vi "SetFPGActrlParams_v2.vi"(4 "Twist Lead":T3={"Twist Lead Num (a0,a1)"=[60.0, 120.0, 120.0], "Twist Lead Den (b0,b1)"=[60.0, 120.0, 120.0]} {"Twist Lead Den (b0,b1)" format="%#_5e"; "Twist Lead Num (a0,a1)" format="%#_5e"}, 5 "Notch":T2={"Bend"={"Notch Num (a0,a1,a2)"=[60.0, 120.0, 120.0], "Notch Den (b0,b1)"=[60.0, 120.0, 120.0]}, "Twist"={"Notch Num (a0,a1,a2)"=[60.0, 120.0, 120.0], "Notch Den (b0,b1)"=[60.0, 120.0, 120.0]}} {"Twist"."Notch Den (b0,b1)" format="%#_5e"; "Twist"."Notch Num (a0,a1,a2)" format="%#_5e"; "Bend"."Notch Den (b0,b1)" format="%#_5e"; "Bend"."Notch Num (a0,a1,a2)" format="%#_5e"}, 6 "Bend Lead":T4={"Bend Lead Num (a1,a2)"=[60.0, 120.0, 120.0], "Bend Lead Den (b0,b1)"=[60.0, 120.0, 120.0]} {"Bend Lead Den (b0,b1)" format="%#_5e"; "Bend Lead Num (a1,a2)" format="%#_5e"}, 7 "Run Controller?":bool, 8 "error in (no error)":errorcluster, 9 "Ki*Ts":T1=[120.0, 60.0, 60.0], 10 "Kp":T5=[10000.0, 10000000.0, 10000000.0] format="%#_5g", 11 "FPGA VI Reference In":T6) -> (0 "error out":errorcluster, 3 "FPGA VI Reference Out":T6)   [LabVIEW 2017]
doc: "Pass parameters to FPGA:\n- Run controller?\n- Kp\n- Ki\n- tau, w0 (lead)\n- LPF_omega"
uses:
  <vilib>/rvi/interface/nirviReadWriteControl/nirviReadWriteControl.xnode
  TypeDefs/FPGA VI Reference.ctl
  FPGA Bitfiles/flexlab_FPGATarget_Tbeam256MAMainVI_XFHOL9u-69o.lvbitx
  NiFpgaLv.dll
  <vilib>/Utility/error.llb/Error Cluster From Error Code.vi
  <vilib>/rvi/errors/niLvFpgaAdjustHostInterfaceError.vi
  TypeDefs/Kp.ctl
  TypeDefs/Ki.ctl
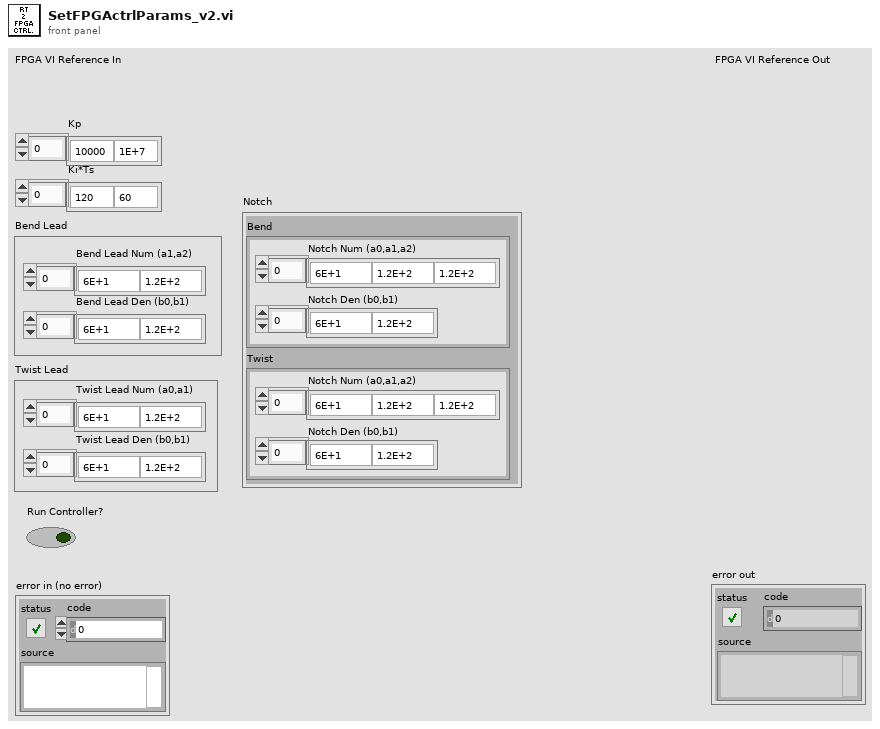
[diagram p1: front panel]
types:
  T1 = typedef "Ki.ctl" = dbl[]
  T2 = cluster{"Bend":cluster{"Notch Num (a0,a1,a2)":T1, "Notch Den (b0,b1)":T1}, "Twist":cluster{"Notch Num (a0,a1,a2)":T1, "Notch Den (b0,b1)":T1}}
  T3 = cluster{"Twist Lead Num (a0,a1)":T1, "Twist Lead Den (b0,b1)":T1}
  T4 = cluster{"Bend Lead Num (a1,a2)":T1, "Bend Lead Den (b0,b1)":T1}
  T5 = typedef "Kp.ctl" = dbl[]
  T6 = typedef "FPGA VI Reference.ctl" = refnum<k20>
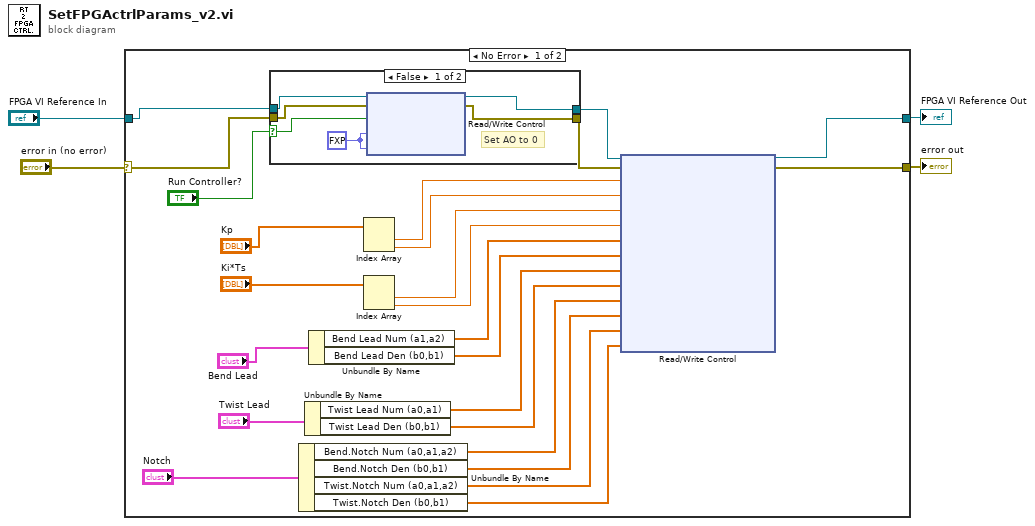
[diagram p0: block diagram]
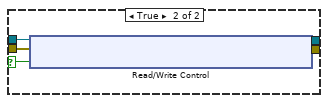
[diagram p2: hidden frame]
diagram:
  n1 = case shown="No Error" "error in (no error)" {
    selector: "error in (no error)" -> [w23 w41]
    tunnel: [w22 w41] -> w3
    tunnel: [w28 w40] -> w1
    tunnel: "FPGA VI Reference In" -> [w25 w40]
    frame No Error {
      n2 = case shown="False" "Run Controller?" {
        selector: "Run Controller?" -> [w32 w35]
        tunnel: w25 -> [w34 w39]
        tunnel: [w30 w38] -> w24
        tunnel: w23 -> [w33 w37]
        tunnel: [w29 w36] -> w10
        frame False {
          w31 = fxp<+/-,26,4> 0.0 ("U_twist [V]")
          # "Set AO to 0"
          n3 = xnode "Read/Write Control"("FPGA VI Reference In"=w34, "error in"=w33, "Run controller?"=w32, "U_twist [V]"=w31, "U_bend [V]"=w31) -> ("FPGA VI Reference Out"=w30:T6, "error out"=w29:errorcluster)
        }
        frame True {
          n4 = xnode "Read/Write Control"("FPGA VI Reference In"=w39, "error in"=w37, "Run controller?"=w35) -> ("FPGA VI Reference Out"=w38:T6, "error out"=w36:errorcluster)
        }
      }
      n5 = Unbundle By Name("Notch") -> ("Bend.Notch Num (a0,a1,a2)"=w8:T1, "Bend.Notch Den (b0,b1)"=w7:T1, "Twist.Notch Num (a0,a1,a2)"=w6:T1, "Twist.Notch Den (b0,b1)"=w5:T1)
      n6 = Unbundle By Name("Twist Lead") -> ("Twist Lead Num (a0,a1)"=w13:T1, "Twist Lead Den (b0,b1)"=w12:T1)
      n7 = Unbundle By Name("Bend Lead") -> ("Bend Lead Num (a1,a2)"=w15:T1, "Bend Lead Den (b0,b1)"=w14:T1)
      n8 = Index Array(array="Kp") -> (element #1=w21:dbl, element #2=w20:dbl)  [unwired: 2 in]
      n9 = Index Array(array="Ki*Ts") -> (element #1=w19:dbl, element #2=w18:dbl)  [unwired: 2 in]
      n10 = xnode "Read/Write Control"("FPGA VI Reference In"=w24, "error in"=w10, "Kp bend"=w21, "Kp twist"=w20, "Ki*Ts bend"=w19, "Ki*Ts twist"=w18, "Bend Lead Numerator"=w15, "Bend Lead Denominator"=w14, "Twist Lead Numerator"=w13, "Twist Lead Denominator"=w12, "Bend Notch Numerator"=w8, "Bend Notch Denominator"=w7, "Twist Notch Numerator"=w6, "Twist Notch Denominator"=w5) -> ("FPGA VI Reference Out"=w28:T6, "error out"=w22:errorcluster)
    }
    frame Error {
    }
  }
  "error out" <- w3
  "FPGA VI Reference Out" <- w1
